vi "P1 Cluster Wrapper.vi"(7 "COM Selector Refs":refnum<vi>[](array[refnum]), 8 "error in(no error)":errorcluster, 9 "P 1 (App) in":T1) -> (0 "error out":errorcluster, 1 "P 1 (App) out":T2)   [LabVIEW 2011]
uses:
  Options Page 1 (App).ctl
  Options Page 1 for display.ctl
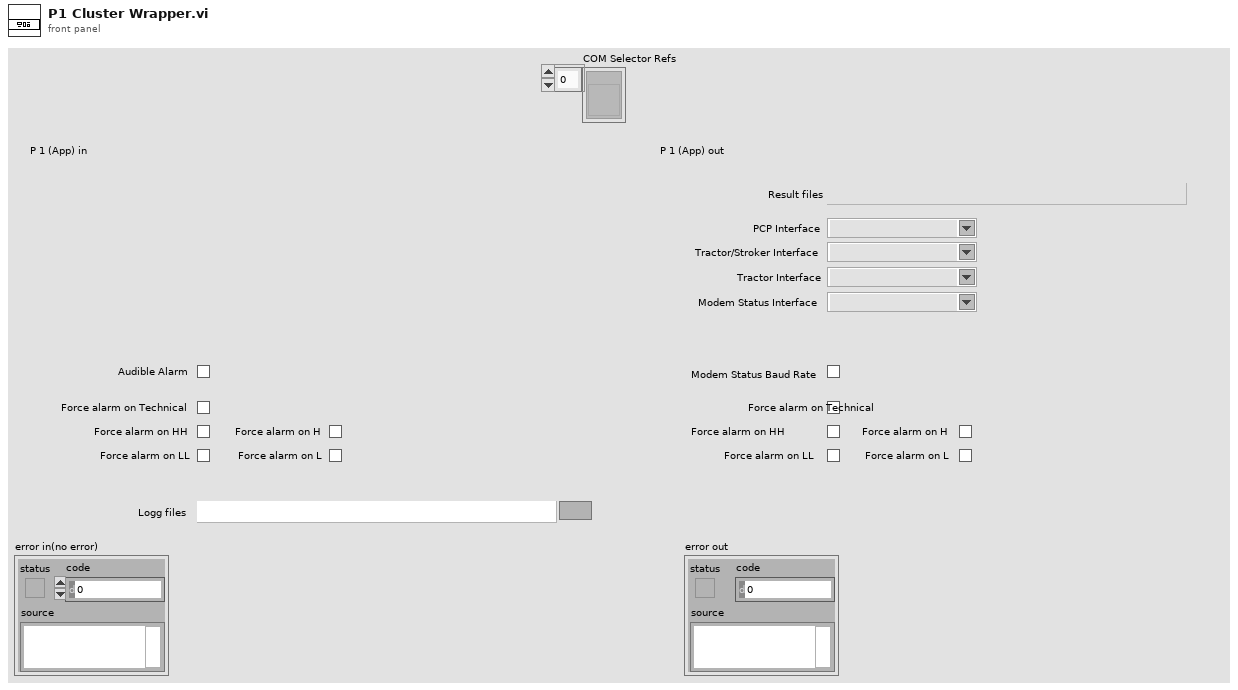
[diagram p1: front panel]
types:
  T1 = typedef "Options Page 1 for display.ctl" = cluster{"Logg files":path, "Audible Alarm":bool, "Force alarm on Technical":bool, "Force alarm on HH":bool, "Force alarm on LL":bool, "Force alarm on H":bool, "Force alarm on L":bool}
  T2 = typedef "Options Page 1 (App).ctl" = cluster{"Result files":path, "PCP Interface":string, "Tractor/Stroker Interface":string, "Tractor Interface":string, "Modem Status Interface":string, "Audible Alarm":bool, "Force alarm on Technical":bool, "Force alarm on HH":bool, "Force alarm on LL":bool, "Force alarm on H":bool, "Force alarm on L":bool}
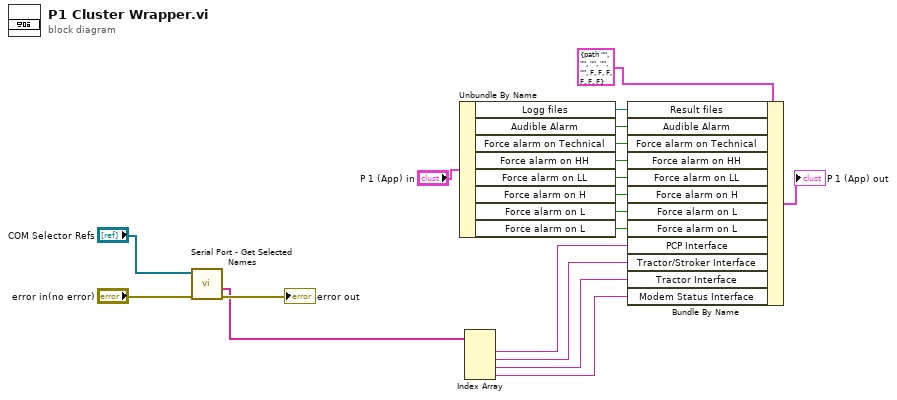
[diagram p0: block diagram]
diagram:
  n1 = call "Serial Port - Get Selected Names.vi"("error in (no error)"="error in(no error)", "Ctrl Refs in"="COM Selector Refs") -> ("error out"=→"error out":errorcluster, "Selected Names"=w2:string[])  [unwired: 8 in]
  n2 = Unbundle By Name("P 1 (App) in") -> ("Logg files"=w16:path, "Audible Alarm"=w15:bool, "Force alarm on Technical"=w14:bool, "Force alarm on HH"=w13:bool, "Force alarm on LL"=w12:bool, "Force alarm on H"=w11:bool, "Force alarm on L"=w10:bool, "Force alarm on L"=w9:bool)
  n3 = Index Array(array=w2) -> (element #1=w8:string, element #2=w7:string, element #3=w6:string, element #4=w5:string)  [unwired: 4 in]
  n4 = Bundle By Name(cluster=T2 {"Result files"=path "", "PCP Interface"="", "Tractor/Stroker Interface"="", "Tractor Interface"="", "Modem Status Interface"="", "Audible Alarm"=FALSE, "Force alarm on Technical"=FALSE, "Force alarm on HH"=FALSE, "Force alarm on LL"=FALSE, "Force alarm on H"=FALSE, "Force alarm on L"=FALSE} ("P 1 (App) out"), "Result files"=w16, "Audible Alarm"=w15, "Force alarm on Technical"=w14, "Force alarm on HH"=w13, "Force alarm on LL"=w12, "Force alarm on H"=w11, "Force alarm on L"=w10, "Force alarm on L"=w9, "PCP Interface"=w8, "Tractor/Stroker Interface"=w7, "Tractor Interface"=w6, "Modem Status Interface"=w5) -> (→"P 1 (App) out":T2)
